vi "Add Update Key Map.vi"(8 "error in (no error)":errorcluster, 9 "Value":string, 10 "Key":string, 11 "Configuration in":refnum<class "Configuration.lvclass">) -> (0 "error out":errorcluster, 3 "Configuration out":refnum<class "Configuration.lvclass">)   [LabVIEW 2023, in "Configuration.lvlib" / "Configuration.lvclass"]
uses:
  Library/Configuration.lvclass
  Library/Configuration.lvclass/Configuration.ctl
  <vilib>/Utility/miscctls.llb/LVMapReplaceAction.ctl
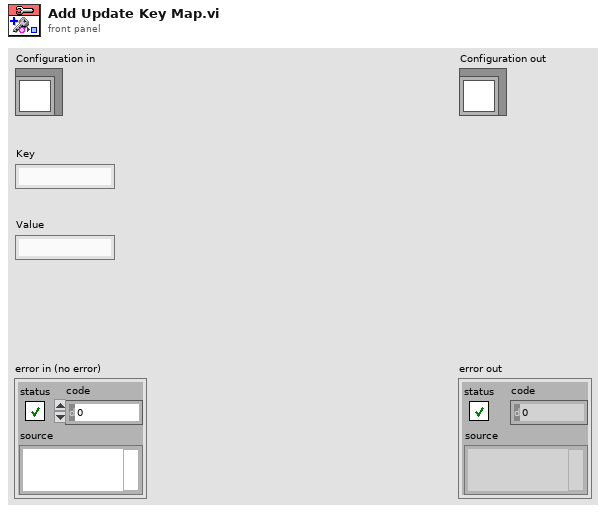
[diagram p1: front panel]
types:
  T1 = typedef "LVMapReplaceAction.ctl" = enum32{"Modify Entry only if found", "Add or Modify Entry", "Delete Entry"}
  T2 = typedef "Configuration.lvlib/Configuration.lvclass/Definitions.ctl" = map{string, T3}
  T3 = typedef "Configuration.lvlib/Configuration.lvclass/Config.ctl" = map{string, string}
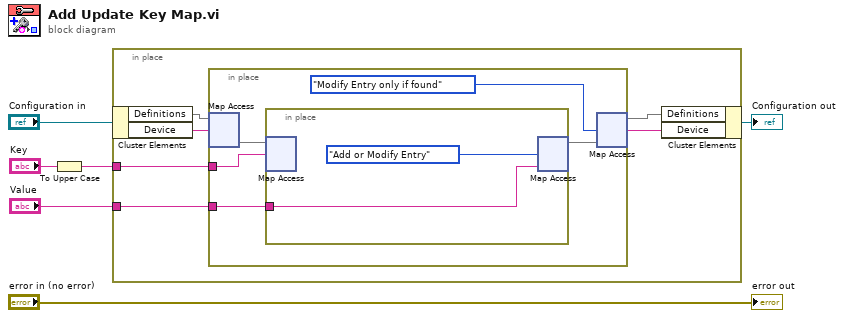
[diagram p0: block diagram]
diagram:
  n1 = To Upper Case(1:"Key") -> (0:w2:string)
  n2 = in-place {
    in-place-border: w2 -> [w8]
    in-place-border: "Value" -> [w7]
    n3 = in-place-cluster #1("Configuration in") -> ("Definitions"=w12:T2, "Device"=w11:string)
    n4 = in-place {
      in-place-border: w8 -> [w13]
      in-place-border: w7 -> [w14]
      n5 = in-place-map #2(w12, w11) -> (w16:T3)  [unwired: 1 in, 1 out]
      n6 = in-place {
        in-place-border: w14 -> [w19]
        n7 = in-place-map #3(w16, w13) -> ()  [unwired: 1 in, 2 out]
        n8 = in-place-map #3(w19, LVMapReplaceAction."Add or Modify Entry" ("action")) -> (w15:T3)  [unwired: 2 out]
      }
      n9 = in-place-map #2(w15, LVMapReplaceAction."Modify Entry only if found" ("action")) -> (w10:T2, w9:string)  [unwired: 1 out]
    }
    n10 = in-place-cluster #1("Definitions"=w10, "Device"=w9) -> (→"Configuration out":refnum<class "Configuration.lvclass">)
  }
  "error out" <- "error in (no error)"
